vi "check_instrument_error.vi"(6 "Mode (Check error from Session)":T1(ring)=enum."Check error from Session", 7 "Attribute":T2={"Identifier"="", "Descriptive Name"="", "Data Type"=enum."Integer 32", "Command"="", "Access"=enum."Read/Write", "Range Table"="", "Read Callback"="", "Write Callback"="", "Supported Models"="", "Instrument Options"="", "Index"=0, "OPC Wait"=FALSE, "No Status Check"=FALSE, "Cache Only"=FALSE}, 8 "error in":errorcluster caption="error in (no error)", 11 "VISA resource name":refnum<visa-resource-name>) -> (0 "error out":errorcluster, 3 "VISA resource name out":refnum<visa-resource-name>)   [LabVIEW 2022 SP3, in "hmp4000_rsidr_core.lvlib"]
uses:
  hmp4000_rsidr_core.lvlib
  type_Attribute.ctl
  type_Attribute_Data_Type.ctl
  type_ReadWriteAccess.ctl
  type_AdditionalFlag_Bits.ctl
  type_Error_Codes.ctl
  Match Regular Expression.xnode
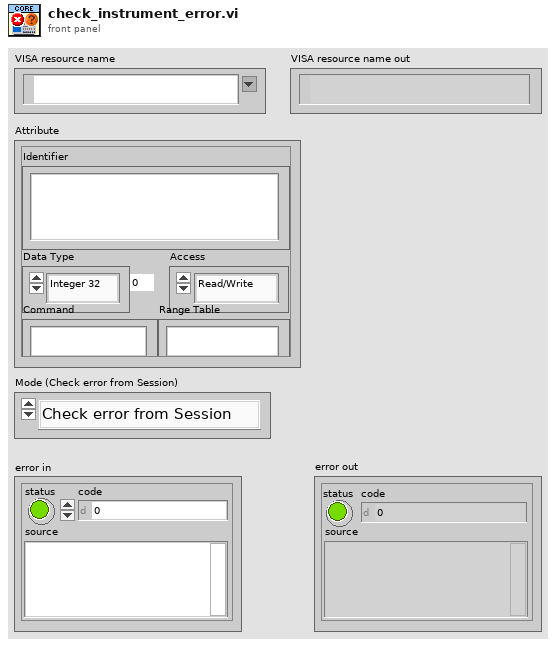
[diagram p1: front panel]
types:
  T1 = enum16{"Check error", "Don't check error", "Check error from Session"}
  T2 = typedef "hmp4000_rsidr_core.lvlib/type_Attribute.ctl" = cluster{"Identifier":string, "Descriptive Name":string, "Data Type":T3, "Command":string, "Access":T4, "Range Table":string, "Read Callback":string, "Write Callback":string, "Supported Models":string, "Instrument Options":string, "Index":i32, "OPC Wait":bool, "No Status Check":bool, "Cache Only":bool}
  T3 = typedef "hmp4000_rsidr_core.lvlib/type_Attribute_Data_Type.ctl" = enum16{"Integer 32", "Double", "String", "Boolean", "None", "Integer 64", "RawString"}
  T4 = typedef "hmp4000_rsidr_core.lvlib/type_ReadWriteAccess.ctl" = enum16{"Read Only", "Write Only", "Read/Write"}
  T5 = typedef "hmp4000_rsidr_core.lvlib/type_AdditionalFlag_Bits.ctl" = enum16{"Send LF after Bin Block", "Junk read with io_clear_buffers.vi", "io_clear_buffers: viClear()", "io_clear_buffers: viFlush()", "<NotUsed1>", "Allow Dbl & Int Bin/Ascii read", "*OPC? in check_instrument_error.vi", "<NotUsed2>", "Smart Enum Matching", "Less Strict RepCaps check", "AssureResponseEndWithLF"}
  T6 = typedef "hmp4000_rsidr_core.lvlib/type_Session_Data.ctl" = cluster{"IDN string":string, "Instrument FW":string, "Instr type":string, "Instr type for err. msg.":string, "Installed Options":string[], "Ignore Error Messages":string, "Logging params":variant, "OPC Timeout":i32, "VISA Timeout":i32, "STB Poll VISA Timeout":i32, "Additional Flags":i32, "Wait Before Read":i32, "Wait Before Write":i32, "Option String Flags":i32, "IO Segment Size":i64, "VISA Access Mode":T7, "Interface Type":T8, "OPC Wait Mode":T9, "Bin Float Number  Format":T10, "Bin Integer Number Format":T11, "Simulate":bool, "VXIcapable":bool, "Duplicate Session":bool, "Add LF to Write":bool, "Logging":bool, "Fast Sweep":bool, "Query Instrument Status":bool, "Check Range":bool, "Check Options":bool}
  T7 = typedef "hmp4000_rsidr_core.lvlib/type_VisaAccessMode.ctl" = u16
  T8 = typedef "hmp4000_rsidr_core.lvlib/type_InterfaceType.ctl" = enum16{"Unknown", "GPIB", "VXI", "GPIB_VXI", "ASRL", "PXI", "TCPIP", "USB", "SOCKET"}
  T9 = typedef "hmp4000_rsidr_core.lvlib/type_OPC_Wait_Mode.ctl" = enum16{"STBpolling", "STBpollingSlow", "STBpollingSuperSlow", "ServiceRequest", "OPCquery"}
  T10 = typedef "hmp4000_rsidr_core.lvlib/type_Binary_Float_Number_Format.ctl" = enum16{"Float_4_Bytes_Swapped", "Float_4_Bytes", "Double_8_Bytes_Swapped", "Double_8_Bytes"}
  T11 = typedef "hmp4000_rsidr_core.lvlib/type_Binary_Integer_Number_Format.ctl" = enum16{"Int32_4_Bytes_Swapped", "Int32_4 Bytes", "Int16_2_Bytes_Swapped", "Int16_2_Bytes"}
  T12 = typedef "hmp4000_rsidr_core.lvlib/type_Error_Codes.ctl" = enum16{"No_error", "VISA_err_ResourceNotFound", "VISA_err_Timeout", "VISA_warn_MoreDataAvailable", "RS_err_MissingCallback", "RS_err_InvalidAttribute", "RS_err_InvalidValue", "RS_err_UnknownResource", "RS_err_AlreadyInitialized", "RS_err_InstrumentStatus", "RS_err_BadRepCapName", "RS_err_TypesMismatch", "RS_err_ValueNotSupported", "RS_err_InvalidRngTable", "RS_err_IDqueryFail", "RS_err_UnexpResponse", "VISA_warn_ConfigNotLoaded", "RS_err_AttributeNotReadable", "RS_err_AttributeNotWritable", "RS_err_InstrumentType", "RS_err_InstrumentOption", "VISA_err_InvalidSize", "RS_err_ReliabilityIndicator", "VISA_warn_UnknownStatus", "VISA_warn_TermCharRead", "VISA_err_IO_error", "RS_err_FunctionNotSupported", "VISA_warn_QueueEmpty"}
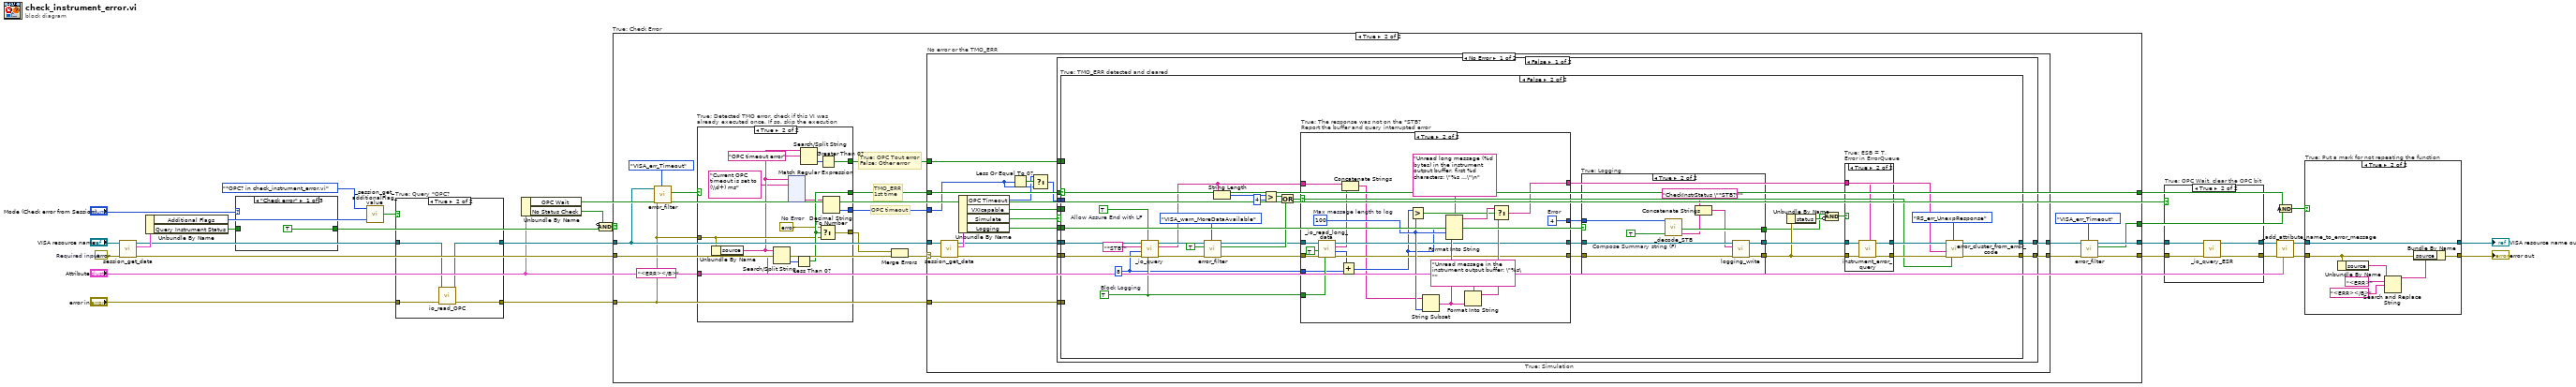
[diagram p0: block diagram]
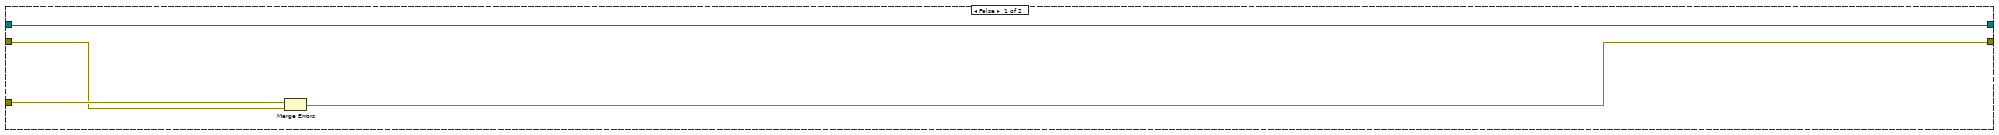
[diagram p5: hidden frame]
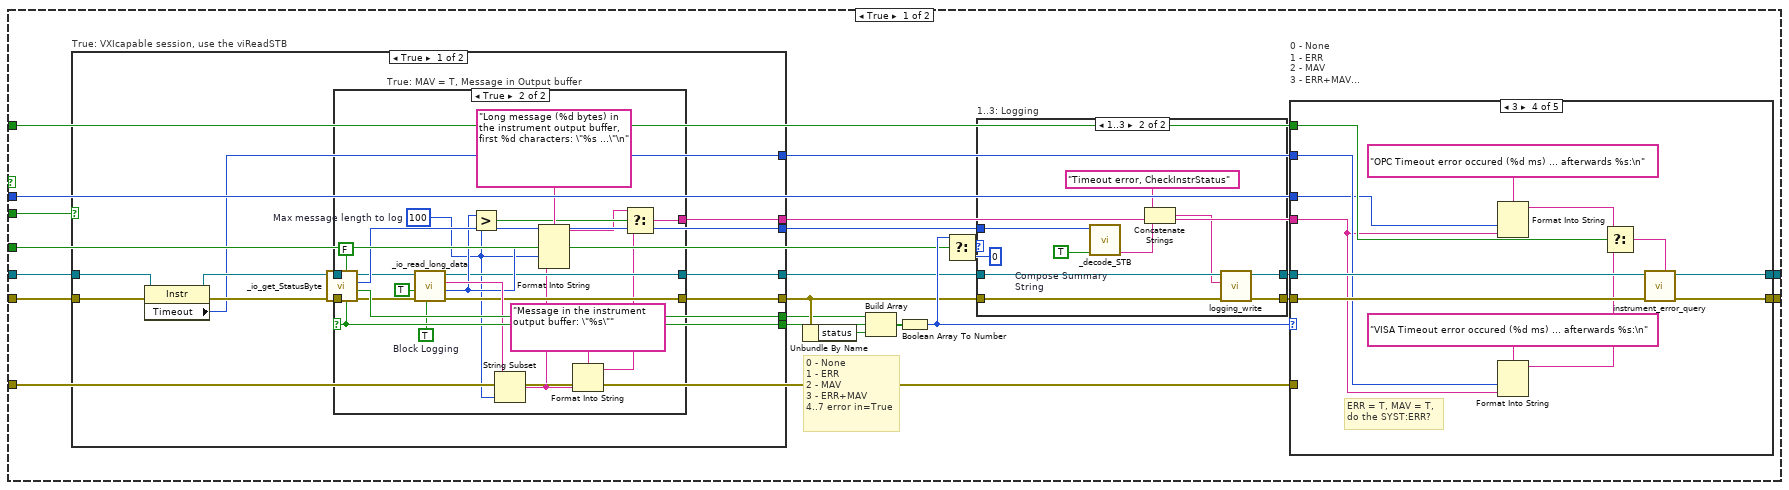
[diagram p7: hidden frame]
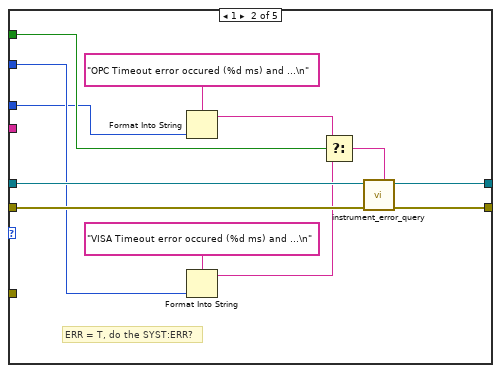
[diagram p9: hidden frame]
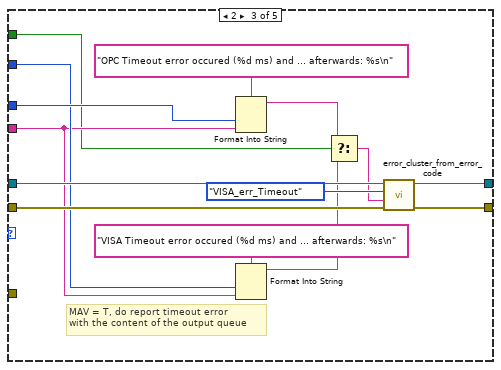
[diagram p10: hidden frame]
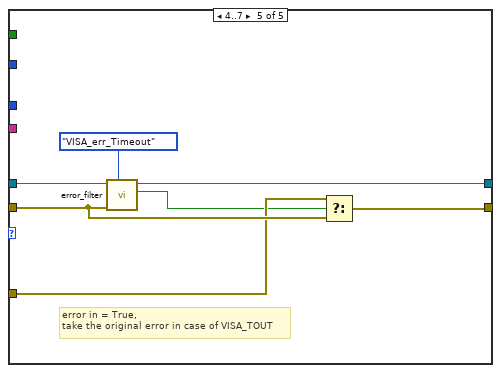
[diagram p11: hidden frame]
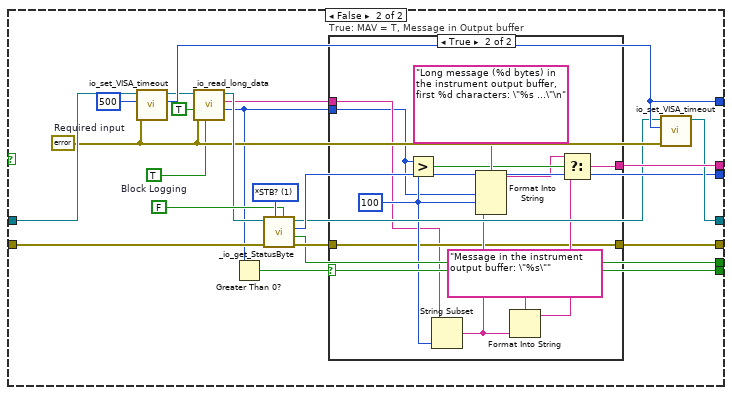
[diagram p14: hidden frame]
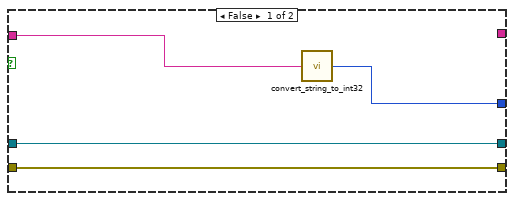
[diagram p16: hidden frame]
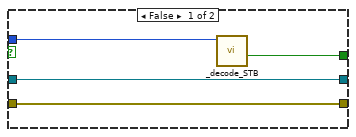
[diagram p18: hidden frame]
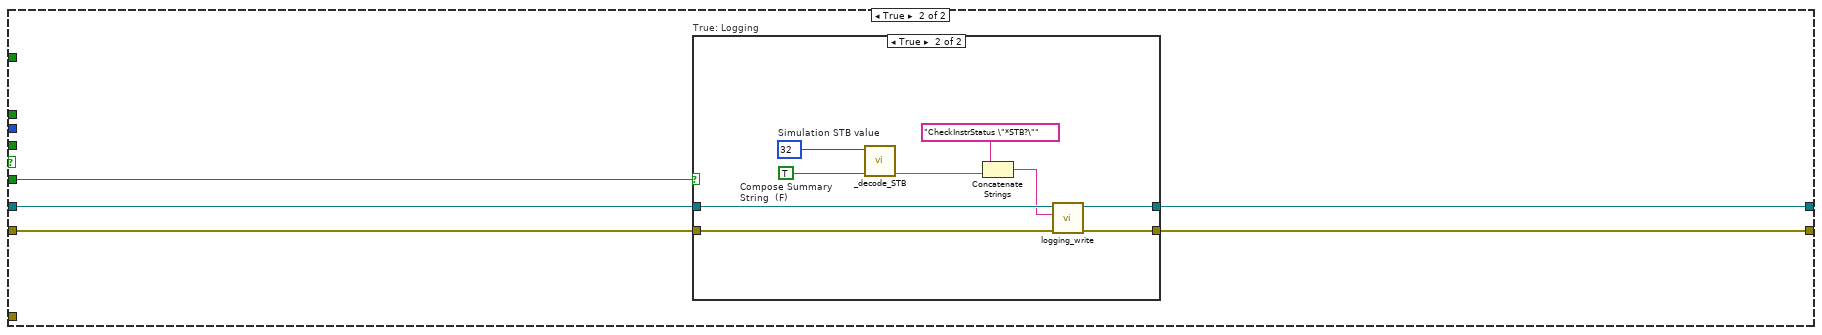
[diagram p19: hidden frame]
diagram:
  w20 = errorcluster {"status"=FALSE, "code"=0, "source"=""}  # Required input
  n1 = call "session_get_data.vi"("error in"=w20, "VISA resource name"="VISA resource name") -> ("error out"=w16:errorcluster, "Session User Data out"=w21:T6, "VISA resource name out"=w18:refnum<visa-resource-name>)  [unwired: 6 in, 1 out]
  n2 = Unbundle By Name(w21) -> ("Additional Flags"=w4:i32, "Query Instrument Status"=w19:bool)
  n3 = case shown="\"Check error\"" "Mode (Check error from Session)" {
    tunnel: [TRUE ("Boolean Out") _ w31] -> w28
    tunnel: w19 -> [_ _ w31]
    frame "Check error" {
    }
    frame "Don't check error" {
    }
    frame "Check error from Session" {
    }
  }
  n4 = call "_session_get_additionalFlag_value.vi"("AdditionalFlags value in"=w4, "AdditionalFlag bit"=type_AdditionalFlag_Bits."*OPC? in check_instrument_error.vi") -> ("AdditionalFlag bit value out"=w5:bool)  [unwired: 3 in]
  n5 = case "True: Query *OPC?" shown="True" w5 {
    tunnel: w18 -> [w32 w35]
    tunnel: [w32 w34] -> w17
    tunnel: "error in" -> [w33 w37]
    tunnel: [w33 w36] -> w14
    frame False {
    }
    frame True {
      n6 = call "io_read_OPC.vi"("error in"=w37, "VISA resource name"=w35) -> ("error out"=w36:errorcluster, "VISA resource name out"=w34:refnum<visa-resource-name>)  [unwired: 7 in, 1 out]
    }
  }
  n7 = Unbundle By Name("Attribute") -> ("OPC Wait"=w26:bool, "No Status Check"=w23:bool)
  n8 = Compound Arithmetic op=AND(invert w23, w28) -> (w27:bool)
  n9 = case "True: Check Error" shown="True" w27 {
    tunnel: [w41 w45] -> w24
    tunnel: [w39 w46] -> w25
    tunnel: w17 -> [w41 w56]
    tunnel: w16 -> [w38 w57]
    tunnel: w14 -> [w40 w53]
    tunnel: [_ w50] -> w7
    tunnel: [_ w44] -> w6
    frame False {
      n10 = Merge Errors(w40, w38) -> (w39:errorcluster)
    }
    frame True {
      # "OPC timeout"
      # "True: OPC Tout error\nFalse: Other error"
      # "TMO_ERR\n1st time"
      n11 = call "error_filter.vi"("Error Enum in"=type_Error_Codes."VISA_err_Timeout", "error in"=w53, "VISA resource name"=w56) -> ("Code Detected"=w54:bool)  [unwired: 6 in, 2 out]
      n12 = case "True: Detected TMO error, check if this VI was\nalready executed once. If so, skip the execution" shown="True" w54 {
        tunnel: w53 -> [w59 w69]
        tunnel: [w59 w71] -> w52
        tunnel: [_ w70] -> w50
        tunnel: "<ERR></B>" ("search string/char (-)") -> [_ w67]
        tunnel: [_ w65] -> w43
        tunnel: [_ w61] -> w42
        frame False {
        }
        frame True {
          w68 = errorcluster {"status"=FALSE, "code"=0, "source"=""}  # No Error
          n13 = Unbundle By Name(w69) -> ("source"=w63:string)
          n14 = Search/Split String(string=w63, search string/char (-)=w67) -> (offset of match=w72:i32)  [unwired: 1 in, 2 out]
          n15 = xnode "Match Regular Expression"("input string"=w63, "regular expression"="Current OPC timeout is set to (\\d+) ms") -> ("submatch 1"=w62:string)  [unwired: 4 in, 5 out]
          n16 = Less Than 0?(x=w72) -> (x < 0?=w70:bool)
          n17 = Search/Split String(string=w63, search string/char (-)="OPC timeout error") -> (offset of match=w66:i32)  [unwired: 1 in, 2 out]
          n18 = Select(t=w68, s=w70, f=w69) -> (s? t:f=w71:errorcluster)
          n19 = Greater Than 0?(x=w66) -> (x > 0?=w65:bool)
          n20 = Decimal String To Number(string=w62) -> (number=w61:i32)  [unwired: 2 in, 1 out]
        }
      }
      n21 = Merge Errors(w52, w57) -> (w55:errorcluster)
      n22 = case "No error or the TMO_ERR" shown="No Error" w55 {
        selector: w55 -> [w202 w461]
        tunnel: [w207 w462] -> w47
        tunnel: [w208 w461] -> w48
        tunnel: w56 -> [w206 w462]
        tunnel: w50 -> [w201 _]
        tunnel: w53 -> [w200 _]
        tunnel: w43 -> [w197 _]
        tunnel: w42 -> [w193 _]
        frame No Error {
          n23 = call "session_get_data.vi"("error in"=w202, "VISA resource name"=w206) -> ("error out"=w204:errorcluster, "Session User Data out"=w205:T6, "VISA resource name out"=w203:refnum<visa-resource-name>)  [unwired: 6 in, 1 out]
          n24 = Unbundle By Name(w205) -> ("OPC Timeout"=w194:i32, "VXIcapable"=w196:bool, "Simulate"=w199:bool, "Logging"=w198:bool)
          n25 = Less Or Equal To 0?(x=w193) -> (x <= 0?=w195:bool)
          n26 = Select(t=w194, s=w195, f=w193) -> (s? t:f=w192:i32)
          n27 = case "True: Simulation" shown="False" w199 {
            tunnel: [w213 w447] -> w208
            tunnel: [w214 w446] -> w207
            tunnel: w204 -> [w217 w449]
            tunnel: w203 -> [w218 w448]
            tunnel: w201 -> [w216 _]
            tunnel: w196 -> [w215 _]
            tunnel: w200 -> [w212 _]
            tunnel: w198 -> [w211 w445]
            tunnel: w192 -> [w210 _]
            tunnel: w197 -> [w209 _]
            frame False {
              n28 = case "True: TMO_ERR detected and cleared" shown="False" w216 {
                tunnel: w218 -> [w228 w397]
                tunnel: w217 -> [w227 w396]
                tunnel: [w224 w370] -> w214
                tunnel: [w223 w371] -> w213
                tunnel: w215 -> [w226 _]
                tunnel: w212 -> [w221 _]
                tunnel: w211 -> [w222 w389]
                tunnel: w210 -> [w220 _]
                tunnel: w209 -> [w219 _]
                frame True {
                  # "0 - None\n1 - ERR\n2 - MAV\n3 - ERR+MAV\n4..7 error in=True"
                  n29 = case "True: VXIcapable session, use the viReadSTB" shown="True" w226 {
                    tunnel: w228 -> [w304 w352]
                    tunnel: w227 -> [w306 w349]
                    tunnel: [w312 w348] -> w235
                    tunnel: [w310 w338] -> w233
                    tunnel: [w311 w347] -> w232
                    tunnel: [w309 w346] -> w238
                    tunnel: [w308 w345] -> w236
                    tunnel: [w307 w344] -> w237
                    tunnel: [w302 w343] -> w225
                    frame True {
                      n30 = property on="Property Node" class="Instr"(reference=w304, error in=w306) -> (reference out=w303:refnum<visa-resource-name>, error out=w305:errorcluster, "Timeout"=w302:u32)
                      n31 = call "_io_get_StatusByte.vi"("Block Setting of VISA Timeout for viReadSTB"=FALSE, "error in"=w305, "VISA resource name"=w303) -> ("error out"=w313:errorcluster, "Error"=w311:bool, "STB returned"=w307:u16, "VISA resource name out"=w314:refnum<visa-resource-name>, "MAV"=w310:bool)  [unwired: 3 in, 1 out]
                      n32 = case "True: MAV = T, Message in Output buffer" shown="True" w310 {
                        tunnel: w313 -> [w316 w332]
                        tunnel: w314 -> [w315 w330]
                        tunnel: [w316 w326] -> w312
                        tunnel: [w315 w327] -> w308
                        tunnel: [_ w319] -> w309
                        frame False {
                        }
                        frame True {
                          w318 = u32 100  # Max message length to log
                          w331 = TRUE  # Block Logging
                          n33 = call "_io_read_long_data.vi"("Block Logging (F)"=w331, "error in"=w332, "Trim Response End (T)"=TRUE, "VISA resource name"=w330) -> ("error out"=w326:errorcluster, "Read bytes count"=w328:u32, "Read buffer"=w329:string, "VISA resource name out"=w327:refnum<visa-resource-name>)  [unwired: 4 in]
                          n34 = Greater?(x=w328, y=w318) -> (0:w322:bool)
                          n35 = String Subset(string=w329, length (rest)=w318) -> (substring=w324:string)  [unwired: 1 in]
                          n36 = Format Into String(format string="Long message (%d bytes) in the instrument output buffer, first %d characters: \"%s ...\"\n", w328, w318, w324) -> (resulting string=w321:string)  [unwired: 2 in, 1 out]
                          n37 = Format Into String(format string="Message in the instrument output buffer: \"%s\"", w324) -> (resulting string=w320:string)  [unwired: 2 in, 1 out]
                          n38 = Select(t=w321, s=w322, f=w320) -> (s? t:f=w319:string)
                        }
                      }
                    }
                    frame False {
                      w334 = TRUE  # Block Logging
                      w339 = errorcluster {"status"=FALSE, "code"=0, "source"=""}  # Required input
                      w350 = u16 1 items=["viReadSTB", "*STB?"] ("Method (viReadSTB)")
                      n39 = call "io_set_VISA_timeout.vi"("error in"=w339, "VISA Timeout"=u32 500, "VISA resource name"=w352) -> ("Old VISA Timeout"=w343:u32, "VISA resource name out"=w341:refnum<visa-resource-name>)  [unwired: 6 in, 1 out]
                      n40 = call "_io_read_long_data.vi"("Block Logging (F)"=w334, "error in"=w339, "Trim Response End (T)"=TRUE, "VISA resource name"=w341) -> ("Read bytes count"=w336:u32, "Read buffer"=w337:string, "VISA resource name out"=w340:refnum<visa-resource-name>)  [unwired: 4 in, 1 out]
                      n41 = Greater Than 0?(x=w336) -> (x > 0?=w338:bool)
                      n42 = call "_io_get_StatusByte.vi"("Block Setting of VISA Timeout for viReadSTB"=FALSE, "Method (viReadSTB)"=w350, "error in"=w349, "VISA resource name"=w340) -> ("error out"=w353:errorcluster, "Error"=w347:bool, "STB returned"=w344:u16, "VISA resource name out"=w335:refnum<visa-resource-name>)  [unwired: 2 in, 2 out]
                      n43 = case "True: MAV = T, Message in Output buffer" shown="True" w338 {
                        tunnel: w353 -> [w354 w357]
                        tunnel: [w354 w357] -> w348
                        tunnel: [_ w358] -> w346
                        tunnel: w337 -> [_ w356]
                        tunnel: w336 -> [_ w355]
                        frame False {
                        }
                        frame True {
                          w365 = u32 100 ("y")
                          n44 = Greater?(x=w355, y=w365) -> (0:w361:bool)
                          n45 = String Subset(string=w356, length (rest)=w365) -> (substring=w363:string)  [unwired: 1 in]
                          n46 = Format Into String(format string="Long message (%d bytes) in the instrument output buffer, first %d characters: \"%s ...\"\n", w355, w365, w363) -> (resulting string=w360:string)  [unwired: 2 in, 1 out]
                          n47 = Format Into String(format string="Message in the instrument output buffer: \"%s\"", w363) -> (resulting string=w359:string)  [unwired: 2 in, 1 out]
                          n48 = Select(t=w360, s=w361, f=w359) -> (s? t:f=w358:string)
                        }
                      }
                      n49 = call "io_set_VISA_timeout.vi"("error in"=w339, "VISA Timeout"=w343, "VISA resource name"=w335) -> ("VISA resource name out"=w345:refnum<visa-resource-name>)  [unwired: 6 in, 2 out]
                    }
                  }
                  n50 = Unbundle By Name(w235) -> ("status"=w231:bool)
                  n51 = Build Array(w232, w233, w231) -> (w230:bool[])
                  n52 = Boolean Array To Number(Boolean array=w230) -> (number=w241:u32)
                  n53 = Select(t=w241, s=w222, f=u32 0) -> (s? t:f=w234:u32)
                  n54 = case "1..3: Logging" shown="1..3" w234 {
                    tunnel: w235 -> [w291 w299]
                    tunnel: [w291 w298] -> w240
                    tunnel: [w290 w297] -> w239
                    tunnel: w236 -> [w290 w296]
                    tunnel: w237 -> [_ w293]
                    frame Default {
                    }
                    frame 1..3 {
                      w300 = TRUE  # Compose Summary String
                      n55 = call "_decode_STB.vi"("Compose Summary string (F)"=w300, "STB in"=w293) -> ("Summary string"=w292:string)  [unwired: 6 in, 3 out]
                      n56 = Concatenate Strings("Timeout error, CheckInstrStatus" ("String to write"), w292) -> (w294:string)
                      n57 = call "logging_write.vi"("error in"=w299, "String to write"=w294, "VISA resource name"=w296) -> ("error out"=w298:errorcluster, "VISA resource name out"=w297:refnum<visa-resource-name>)  [unwired: 7 in]
                    }
                  }
                  n58 = case "0 - None\n1 - ERR\n2 - MAV\n3 - ERR+MAV\n4..7 error in=True" shown="3" w241 {
                    tunnel: w221 -> [w242 _ _ _ w284]
                    tunnel: [w242 w255 w265 w282 w286] -> w223
                    tunnel: w239 -> [w243 w252 w267 w279 w288]
                    tunnel: [w243 w254 w269 w281 w287] -> w224
                    tunnel: w240 -> [_ w251 w266 w278 w285]
                    tunnel: w238 -> [_ _ w260 w270 _]
                    tunnel: w225 -> [_ w250 w261 w277 _]
                    tunnel: w220 -> [_ w247 w263 w274 _]
                    tunnel: w219 -> [_ w249 w257 w276 _]
                    frame 0, Default {
                      # "ERR = F, MAV = F, pass the TMO_ERR forward"
                    }
                    frame 1 {
                      # "ERR = T, do the SYST:ERR?"
                      n59 = Format Into String(format string="OPC Timeout error occured (%d ms) and ...\n" ("Beginning error message string (\"\")"), w247) -> (resulting string=w246:string)  [unwired: 2 in, 1 out]
                      n60 = Format Into String(format string="VISA Timeout error occured (%d ms) and ...\n" ("Beginning error message string (\"\")"), w250) -> (resulting string=w245:string)  [unwired: 2 in, 1 out]
                      n61 = Select(t=w246, s=w249, f=w245) -> (s? t:f=w244:string)
                      n62 = call "instrument_error_query.vi"("Beginning error message string (\"\")"=w244, "error in"=w251, "VISA resource name"=w252) -> ("error out"=w255:errorcluster, "VISA resource name out"=w254:refnum<visa-resource-name>)  [unwired: 5 in, 2 out]
                    }
                    frame 2 {
                      # "MAV = T, do report timeout error\nwith the content of the output queue"
                      n63 = Format Into String(format string="OPC Timeout error occured (%d ms) and ... afterwards: %s\n" ("Beginning error message string (\"\")"), w263, w260) -> (resulting string=w259:string)  [unwired: 2 in, 1 out]
                      n64 = Format Into String(format string="VISA Timeout error occured (%d ms) and ... afterwards: %s\n" ("Beginning error message string (\"\")"), w261, w260) -> (resulting string=w258:string)  [unwired: 2 in, 1 out]
                      n65 = Select(t=w259, s=w257, f=w258) -> (s? t:f=w256:string)
                      n66 = call "error_cluster_from_error_code.vi"("error in"=w266, "Error Message (\"\")"=w256, "Error Enum in"=type_Error_Codes."VISA_err_Timeout", "VISA resource name"=w267) -> ("error out"=w265:errorcluster, "VISA resource name out"=w269:refnum<visa-resource-name>)  [unwired: 6 in]
                    }
                    frame 3 {
                      # "ERR = T, MAV = T,\ndo the SYST:ERR?"
                      n67 = Format Into String(format string="OPC Timeout error occured (%d ms) ... afterwards %s:\n" ("Beginning error message string (\"\")"), w274, w270) -> (resulting string=w273:string)  [unwired: 2 in, 1 out]
                      n68 = Format Into String(format string="VISA Timeout error occured (%d ms) ... afterwards %s:\n" ("Beginning error message string (\"\")"), w277, w270) -> (resulting string=w272:string)  [unwired: 2 in, 1 out]
                      n69 = Select(t=w273, s=w276, f=w272) -> (s? t:f=w271:string)
                      n70 = call "instrument_error_query.vi"("Beginning error message string (\"\")"=w271, "error in"=w278, "VISA resource name"=w279) -> ("error out"=w282:errorcluster, "VISA resource name out"=w281:refnum<visa-resource-name>)  [unwired: 5 in, 2 out]
                    }
                    frame 4..7 {
                      # "error in = True,\ntake the original error in case of VISA_TOUT"
                      n71 = call "error_filter.vi"("Error Enum in"=type_Error_Codes."VISA_err_Timeout", "error in"=w285, "VISA resource name"=w288) -> ("Code Detected"=w283:bool, "VISA resource name out"=w287:refnum<visa-resource-name>)  [unwired: 6 in, 1 out]
                      n72 = Select(t=w284, s=w283, f=w285) -> (s? t:f=w286:errorcluster)
                    }
                  }
                }
                frame False {
                  w366 = TRUE  # Allow Assure End with LF
                  w375 = TRUE  # Block Logging
                  w374 = u32 8 ("byte count (0)")
                  n73 = call "_io_query.vi"("Block Logging (F)"=w375, "Allow Assure End with LF"=w366, "error in"=w396, "Max bytes to read (2048)"=w374, "Write buffer"="*STB?" ("write buffer (\"\")"), "VISA resource name"=w397) -> ("error out"=w384:errorcluster, "Read buffer"=w382:string, "VISA resource name out"=w383:refnum<visa-resource-name>)  [unwired: 2 in, 1 out]
                  n74 = call "error_filter.vi"("Error Enum in"=type_Error_Codes."VISA_warn_MoreDataAvailable", "error in"=w384, "Clear detected code (F)"=TRUE, "VISA resource name"=w383) -> ("error out"=w378:errorcluster, "Code Detected"=w380:bool, "VISA resource name out"=w379:refnum<visa-resource-name>)  [unwired: 5 in]
                  n75 = String Length(string=w382) -> (length=w388:i32)
                  n76 = Greater?(x=w388, y=4) -> (0:w381:bool)
                  n77 = Or(x=w381, y=w380) -> (x .or. y?=w367:bool)
                  n78 = case "True: The response was not on the *STB?\nReport the buffer and query interrupted error" shown="True" w367 {
                    tunnel: [w399 w423] -> w395
                    tunnel: w382 -> [w402 w406]
                    tunnel: [_ w411] -> w369
                    tunnel: w379 -> [w400 w415]
                    tunnel: w378 -> [w401 w414]
                    tunnel: [w400 w413] -> w377
                    tunnel: [w401 w412] -> w376
                    tunnel: w375 -> [_ w410]
                    tunnel: w374 -> [_ w409]
                    frame False {
                      n79 = call "convert_string_to_int32.vi"("String in"=w402) -> ("int32 value out"=w399:i32)  [unwired: 4 in]
                    }
                    frame True {
                      w422 = u32 100  # Max message length to log
                      w423 = 4  # Error
                      n80 = call "_io_read_long_data.vi"("Block Logging (F)"=w410, "error in"=w414, "Trim Response End (T)"=TRUE, "VISA resource name"=w415) -> ("error out"=w412:errorcluster, "Read bytes count"=w408:u32, "Read buffer"=w405:string, "VISA resource name out"=w413:refnum<visa-resource-name>)  [unwired: 4 in]
                      n81 = Add(x=w408, y=w409) -> (x+y=w407:u32)
                      n82 = Concatenate Strings(w406, w405) -> (w404:string)
                      n83 = Greater?(x=w407, y=w422) -> (0:w419:bool)
                      n84 = String Subset(string=w404, length (rest)=w422) -> (substring=w417:string)  [unwired: 1 in]
                      n85 = Format Into String(format string="Unread long message (%d bytes) in the instrument output buffer, first %d characters: \"%s ...\"\n", w407, w422, w417) -> (resulting string=w420:string)  [unwired: 2 in, 1 out]
                      n86 = Format Into String(format string="Unread message in the instrument output buffer: \"%s\"", w417) -> (resulting string=w421:string)  [unwired: 2 in, 1 out]
                      n87 = Select(t=w420, s=w419, f=w421) -> (s? t:f=w411:string)
                    }
                  }
                  n88 = case "True: Logging" shown="True" w389 {
                    tunnel: w376 -> [w433 w444]
                    tunnel: [w433 w443] -> w393
                    tunnel: [w432 w442] -> w394
                    tunnel: w377 -> [w432 w441]
                    tunnel: [w434 w440] -> w391
                    tunnel: w395 -> [w431 w437]
                    frame False {
                      n89 = call "_decode_STB.vi"("STB in"=w431) -> ("Error"=w434:bool)  [unwired: 7 in, 3 out]
                    }
                    frame True {
                      w435 = TRUE  # Compose Summary string (F)
                      n90 = call "_decode_STB.vi"("Compose Summary string (F)"=w435, "STB in"=w437) -> ("Summary string"=w436:string, "Error"=w440:bool)  [unwired: 6 in, 2 out]
                      n91 = Concatenate Strings("CheckInstrStatus \"*STB?\"" ("String to write"), w436) -> (w438:string)
                      n92 = call "logging_write.vi"("error in"=w444, "String to write"=w438, "VISA resource name"=w441) -> ("error out"=w443:errorcluster, "VISA resource name out"=w442:refnum<visa-resource-name>)  [unwired: 7 in]
                    }
                  }
                  n93 = Unbundle By Name(w393) -> ("status"=w392:bool)
                  n94 = Compound Arithmetic op=AND(w391, invert w392) -> (w390:bool)
                  n95 = case "True: ESB = T,\nError in ErrorQueue" shown="True" w390 {
                    tunnel: [w424 w430] -> w373
                    tunnel: [w425 w429] -> w372
                    tunnel: w393 -> [w424 w428]
                    tunnel: w394 -> [w425 w427]
                    tunnel: w369 -> [_ w426]
                    frame False {
                    }
                    frame True {
                      n96 = call "instrument_error_query.vi"("Beginning error message string (\"\")"=w426, "error in"=w428, "VISA resource name"=w427) -> ("error out"=w430:errorcluster, "VISA resource name out"=w429:refnum<visa-resource-name>)  [unwired: 5 in, 2 out]
                    }
                  }
                  n97 = call "error_cluster_from_error_code.vi"("Error Creation Enabled (True)"=w367, "error in"=w373, "Error Message (\"\")"=w369, "Error Enum in"=type_Error_Codes."RS_err_UnexpResponse", "VISA resource name"=w372) -> ("error out"=w371:errorcluster, "VISA resource name out"=w370:refnum<visa-resource-name>)  [unwired: 5 in]
                }
              }
            }
            frame True {
              n98 = case "True: Logging" shown="True" w445 {
                tunnel: w449 -> [w451 w460]
                tunnel: w448 -> [w450 w459]
                tunnel: [w451 w458] -> w447
                tunnel: [w450 w457] -> w446
                frame False {
                }
                frame True {
                  w455 = TRUE  # Compose Summary String  (F)
                  w456 = u16 32  # Simulation STB value
                  n99 = call "_decode_STB.vi"("Compose Summary string (F)"=w455, "STB in"=w456) -> ("Summary string"=w452:string)  [unwired: 6 in, 3 out]
                  n100 = Concatenate Strings("CheckInstrStatus \"*STB?\"" ("String to write"), w452) -> (w453:string)
                  n101 = call "logging_write.vi"("error in"=w460, "String to write"=w453, "VISA resource name"=w459) -> ("error out"=w458:errorcluster, "VISA resource name out"=w457:refnum<visa-resource-name>)  [unwired: 7 in]
                }
              }
            }
          }
        }
        frame Error {
          # "Communication error or error\nchecking turned off"
        }
      }
      n102 = call "error_filter.vi"("Error Enum in"=type_Error_Codes."VISA_err_Timeout", "error in"=w48, "VISA resource name"=w47) -> ("error out"=w46:errorcluster, "Code Detected"=w44:bool, "VISA resource name out"=w45:refnum<visa-resource-name>)  [unwired: 6 in]
    }
  }
  n103 = case "True: OPC Wait, clear the OPC bit" shown="True" w26 {
    tunnel: w25 -> [w464 w468]
    tunnel: w24 -> [w463 w467]
    tunnel: [w464 w466] -> w11
    tunnel: [w463 w465] -> w2
    frame False {
    }
    frame True {
      n104 = call "_io_query_ESR.vi"("error in"=w468, "VISA resource name"=w467) -> ("error out"=w466:errorcluster, "VISA resource name out"=w465:refnum<visa-resource-name>)  [unwired: 7 in, 1 out]
    }
  }
  n105 = call "_add_attribute_name_to_error_message.vi"("Attribute"="Attribute", "error in"=w11, "VISA resource name"=w2) -> ("error out"=w10:errorcluster, "VISA resource name out"=w1:refnum<visa-resource-name>)  [unwired: 6 in, 1 out]
  n106 = And(x=w7, y=w6) -> (x .and. y?=w9:bool)
  n107 = case "True: Put a mark for not repeating the function" shown="True" w9 {
    tunnel: w10 -> [w470 w472]
    tunnel: w1 -> [w469 w474]
    tunnel: [w469 w474] -> w13
    tunnel: [w470 w473] -> w12
    frame False {
    }
    frame True {
      n108 = Unbundle By Name(w472) -> ("source"=w476:string)
      n109 = Search and Replace String(input string=w476, search string="<ERR>", replace string="<ERR></B>" ("replace string (\"\")")) -> (result string=w471:string)  [unwired: 5 in, 3 out]
      n110 = Bundle By Name(cluster=w472, "source"=w471) -> (w473:errorcluster)
    }
  }
  "error out" <- w12
  "VISA resource name out" <- w13
